vi "franch_frame_correction.vi"(9 "Frame Offest":i32, 11 "Input Signal":cdb[](array[numeric])) -> (3 "Frame-Synched Signal":cdb[](array[numeric]))   [LabVIEW 2012]
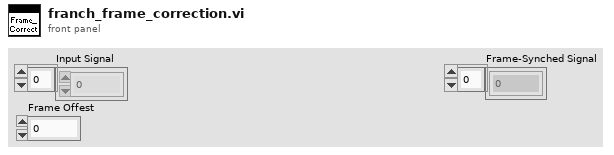
[diagram p1: front panel]
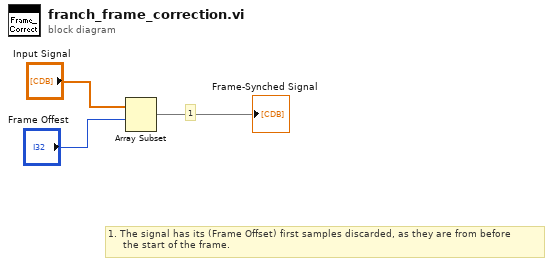
[diagram p0: block diagram]
diagram:
  # "1. The signal has its (Frame Offset) first samples discarded, as they are from before \n     the start of the frame."
  # "1"
  n1 = Array Subset(array="Input Signal", index="Frame Offest") -> (→"Frame-Synched Signal":cdb[])  [unwired: 1 in]
